vi "Init.vi"(0 "ClassReaderNative in":refnum<class "ClassReaderNative.lvclass">, 1 "LvClassRef":refnum<vi>, 5 "error in (no error)":errorcluster) -> (14 "ClassReaderNative out":refnum<class "ClassReaderNative.lvclass">, 19 "error out":errorcluster)   [LabVIEW 2012, in "ClassReaderNative.lvclass"]
uses:
  <resource>/Framework/Providers/Open_GDS/ClassProviders/Provider_LvNativeClass/ClassReaderNative_class/ClassReaderNative.lvclass
  <resource>/Framework/Providers/Open_GDS/ClassProviders/Provider_LvNativeClass/ClassReaderNative_class/ClassReaderNative.lvclass/ClassReaderNative.ctl
  <resource>/Framework/Providers/Open_GDS/ClassProviders/Provider_BaseClassInterface/ClassReader_class/ClassReader.lvclass
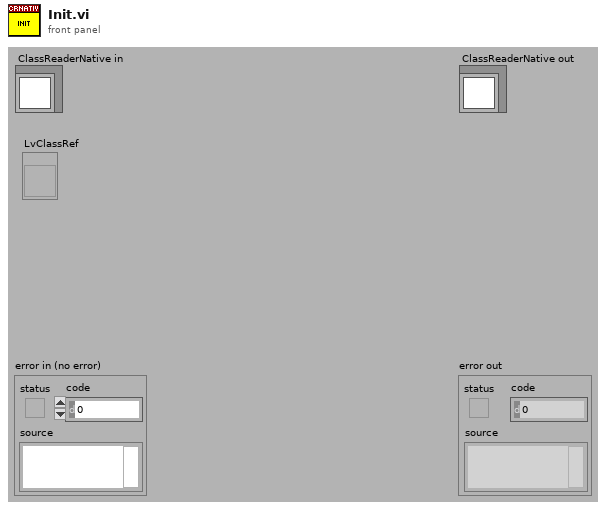
[diagram p1: front panel]
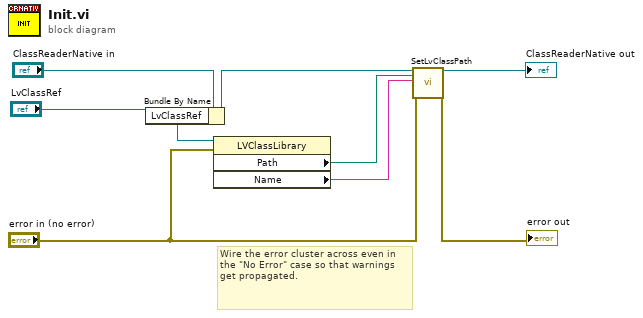
[diagram p0: block diagram]
diagram:
  # "Wire the error cluster across even in the \"No Error\" case so that warnings get propagated."
  n1 = Bundle By Name(cluster="ClassReaderNative in", "LvClassRef"="LvClassRef") -> (w3:refnum<class "ClassReaderNative.lvclass">)
  n2 = property class="LVClassLibrary"(reference="LvClassRef", error in="error in (no error)") -> ("Path"=w2:path, "Name"=w1:string)  [unwired: 2 out]
  n3 = call <resource>:"SetLvClassPath.vi"("reference in"=w3, "ClassPath"=w2, "ClassName"=w1, "error in (no error)"="error in (no error)") -> ("reference out"=→"ClassReaderNative out":refnum<class "ClassReaderNative.lvclass">, "error out"=→"error out":errorcluster)  [unwired: 14 in]
